vi "SPS-Variablen_nach_Cluster.vi"(8 "Fehler in":errorcluster, 11 "Cluster in":T2={"Initialisierung"={"Online?"=FALSE, "Grundpfad"=path "", "Kamera Oben"="", "IP-Adresse Flüssiglinse"="", "Flüssiglinse"=refnum, "Kamera Unten"="", "IP-Adresse SPS"="", "SPS-Verbindung"={"TCP Connection Ref"=refnum, "IP address"="", "timeout ms"=5000, "Connected?"=FALSE, "PLC Type"=enum."S7 1200", "Rack S7 400"=0, "Slot S7 400"=0, "PDU Size"=0, "connection semaphore"=refnum}, "IP-Adresse Lichtgitter"="", "Lichtgitter"=refnum, "Skalierungsfaktor"=0.0, "Bilder Oben"=[], "Bild Unten"=refnum, "Bild Ausschnitt Unten"=refnum}, "Einstellungen"={"Gesamtablauf gestartet"=FALSE, "i. O. Bilder speichern"=FALSE, "Bildspeicherung Offline"=FALSE, "Ausgewähltes Offline-Datum"="", "Ausgewähltes Offline-Teil"="", "Speicherpfad Bilder"=path ""}, "Artikeldaten"={"Artikelnummer"="", "Fertigungsauftrag"="", "Muster ISO"=refnum, "Belichtungszeit Referenzmarken"=0.0, "Fokus Referenzmarken"=0.0, "Belichtungszeit ISO"=0.0, "Fokus ISO"=0.0, "Belichtungszeit Unten"=0.0, "Kontaktanzahl"=0, "Aktueller Kontakt"=0, "Kontaktposition"={"x"=0.0, "y"=0.0}, "Winkel ISO"=0.0, "ISO-Muster nicht vorhanden"=FALSE}, "Werte Kamera Oben"={"Koordinatensystem"={"Punkt x-Achse"={"X"=0.0, "Y"=0.0}, "Ursprung"={"X"=0.0, "Y"=0.0}, "Punkt y-Achse"={"X"=0.0, "Y"=0.0}}, "Position Kontakt"={"x"=0.0, "y"=0.0}, "Winkel Kontakt"=0.0}, "Werte Kamera Unten"={"Prüfung Unten n. i. O."=FALSE}, "Werte Lichtgitter"={"Messwerte Referenzmarken"=[], "Mittelpunkt Referenzmarken"={"x"=0.0, "y"=0.0}, "Messwerte Kontakt"=[], "Offset"={"x"=0.0, "y"=0.0}}, "Rückmeldungen"={"Koordinaten ermittelt"=FALSE, "Vermessung Lichtgitter fertig"=FALSE, "Nachkontrolle Kamera Unten fertig"=FALSE}, "Fehler"={"Referenzen nicht gefunden"=FALSE, "Kontakt nicht gefunden"=FALSE, "Referenzen nicht in Lichtgitter"=FALSE, "Kontakt zu groß"=FALSE, "Kontakt zu klein"=FALSE}, "Statistik"={"Statistiken"=[]}, "Timer"={"Timer Start Position"=0, "Timer Start Lichtgitter"=0, "Timer Start Kamera Unten"=0}}) -> (0 "Fehler out":errorcluster, 1 "SPS OUT":T1, 2 "SPS IN":T10, 3 "Cluster out":T2={"Initialisierung"={"Online?"=FALSE, "Grundpfad"=path "", "Kamera Oben"="", "IP-Adresse Flüssiglinse"="", "Flüssiglinse"=refnum, "Kamera Unten"="", "IP-Adresse SPS"="", "SPS-Verbindung"={"TCP Connection Ref"=refnum, "IP address"="", "timeout ms"=5000, "Connected?"=FALSE, "PLC Type"=enum."S7 1200", "Rack S7 400"=0, "Slot S7 400"=0, "PDU Size"=0, "connection semaphore"=refnum}, "IP-Adresse Lichtgitter"="", "Lichtgitter"=refnum, "Skalierungsfaktor"=0.0, "Bilder Oben"=[], "Bild Unten"=refnum, "Bild Ausschnitt Unten"=refnum}, "Einstellungen"={"Gesamtablauf gestartet"=FALSE, "i. O. Bilder speichern"=FALSE, "Bildspeicherung Offline"=FALSE, "Ausgewähltes Offline-Datum"="", "Ausgewähltes Offline-Teil"="", "Speicherpfad Bilder"=path ""}, "Artikeldaten"={"Artikelnummer"="", "Fertigungsauftrag"="", "Muster ISO"=refnum, "Belichtungszeit Referenzmarken"=0.0, "Fokus Referenzmarken"=0.0, "Belichtungszeit ISO"=0.0, "Fokus ISO"=0.0, "Belichtungszeit Unten"=0.0, "Kontaktanzahl"=0, "Aktueller Kontakt"=0, "Kontaktposition"={"x"=0.0, "y"=0.0}, "Winkel ISO"=0.0, "ISO-Muster nicht vorhanden"=FALSE}, "Werte Kamera Oben"={"Koordinatensystem"={"Punkt x-Achse"={"X"=0.0, "Y"=0.0}, "Ursprung"={"X"=0.0, "Y"=0.0}, "Punkt y-Achse"={"X"=0.0, "Y"=0.0}}, "Position Kontakt"={"x"=0.0, "y"=0.0}, "Winkel Kontakt"=0.0}, "Werte Kamera Unten"={"Prüfung Unten n. i. O."=FALSE}, "Werte Lichtgitter"={"Messwerte Referenzmarken"=[], "Mittelpunkt Referenzmarken"={"x"=0.0, "y"=0.0}, "Messwerte Kontakt"=[], "Offset"={"x"=0.0, "y"=0.0}}, "Rückmeldungen"={"Koordinaten ermittelt"=FALSE, "Vermessung Lichtgitter fertig"=FALSE, "Nachkontrolle Kamera Unten fertig"=FALSE}, "Fehler"={"Referenzen nicht gefunden"=FALSE, "Kontakt nicht gefunden"=FALSE, "Referenzen nicht in Lichtgitter"=FALSE, "Kontakt zu groß"=FALSE, "Kontakt zu klein"=FALSE}, "Statistik"={"Statistiken"=[]}, "Timer"={"Timer Start Position"=0, "Timer Start Lichtgitter"=0, "Timer Start Kamera Unten"=0}})   [LabVIEW 2024]
doc: "Bündelt die Globalen Variablen von der SPS in Cluster und gibt diese aus."
uses:
  Cluster_SPS_IN.ctl
  Cluster.ctl
  Kontaktmontagemodul.exe/1abvi3w/vi.lib/userDefined/High Color/IMAQdx.ctl
  Kontaktmontagemodul.exe/1abvi3w/vi.lib/DATA AHEAD/SP7/typedefs/S7 Connection.ctl
  Kontaktmontagemodul.exe/1abvi3w/vi.lib/DATA AHEAD/SP7/typedefs/PLC Type.ctl
  Kontaktmontagemodul.exe/1abvi3w/vi.lib/vision/Image Controls.llb/IMAQ Image.ctl
  Koordinatensystem.ctl
  Statistik.ctl
  Cluster_SPS_OUT.ctl
  Globale Variablen.vi
  Kontaktmontagemodul.exe/1abvi3w/vi.lib/DATA AHEAD/SP7/SP7.lvlib
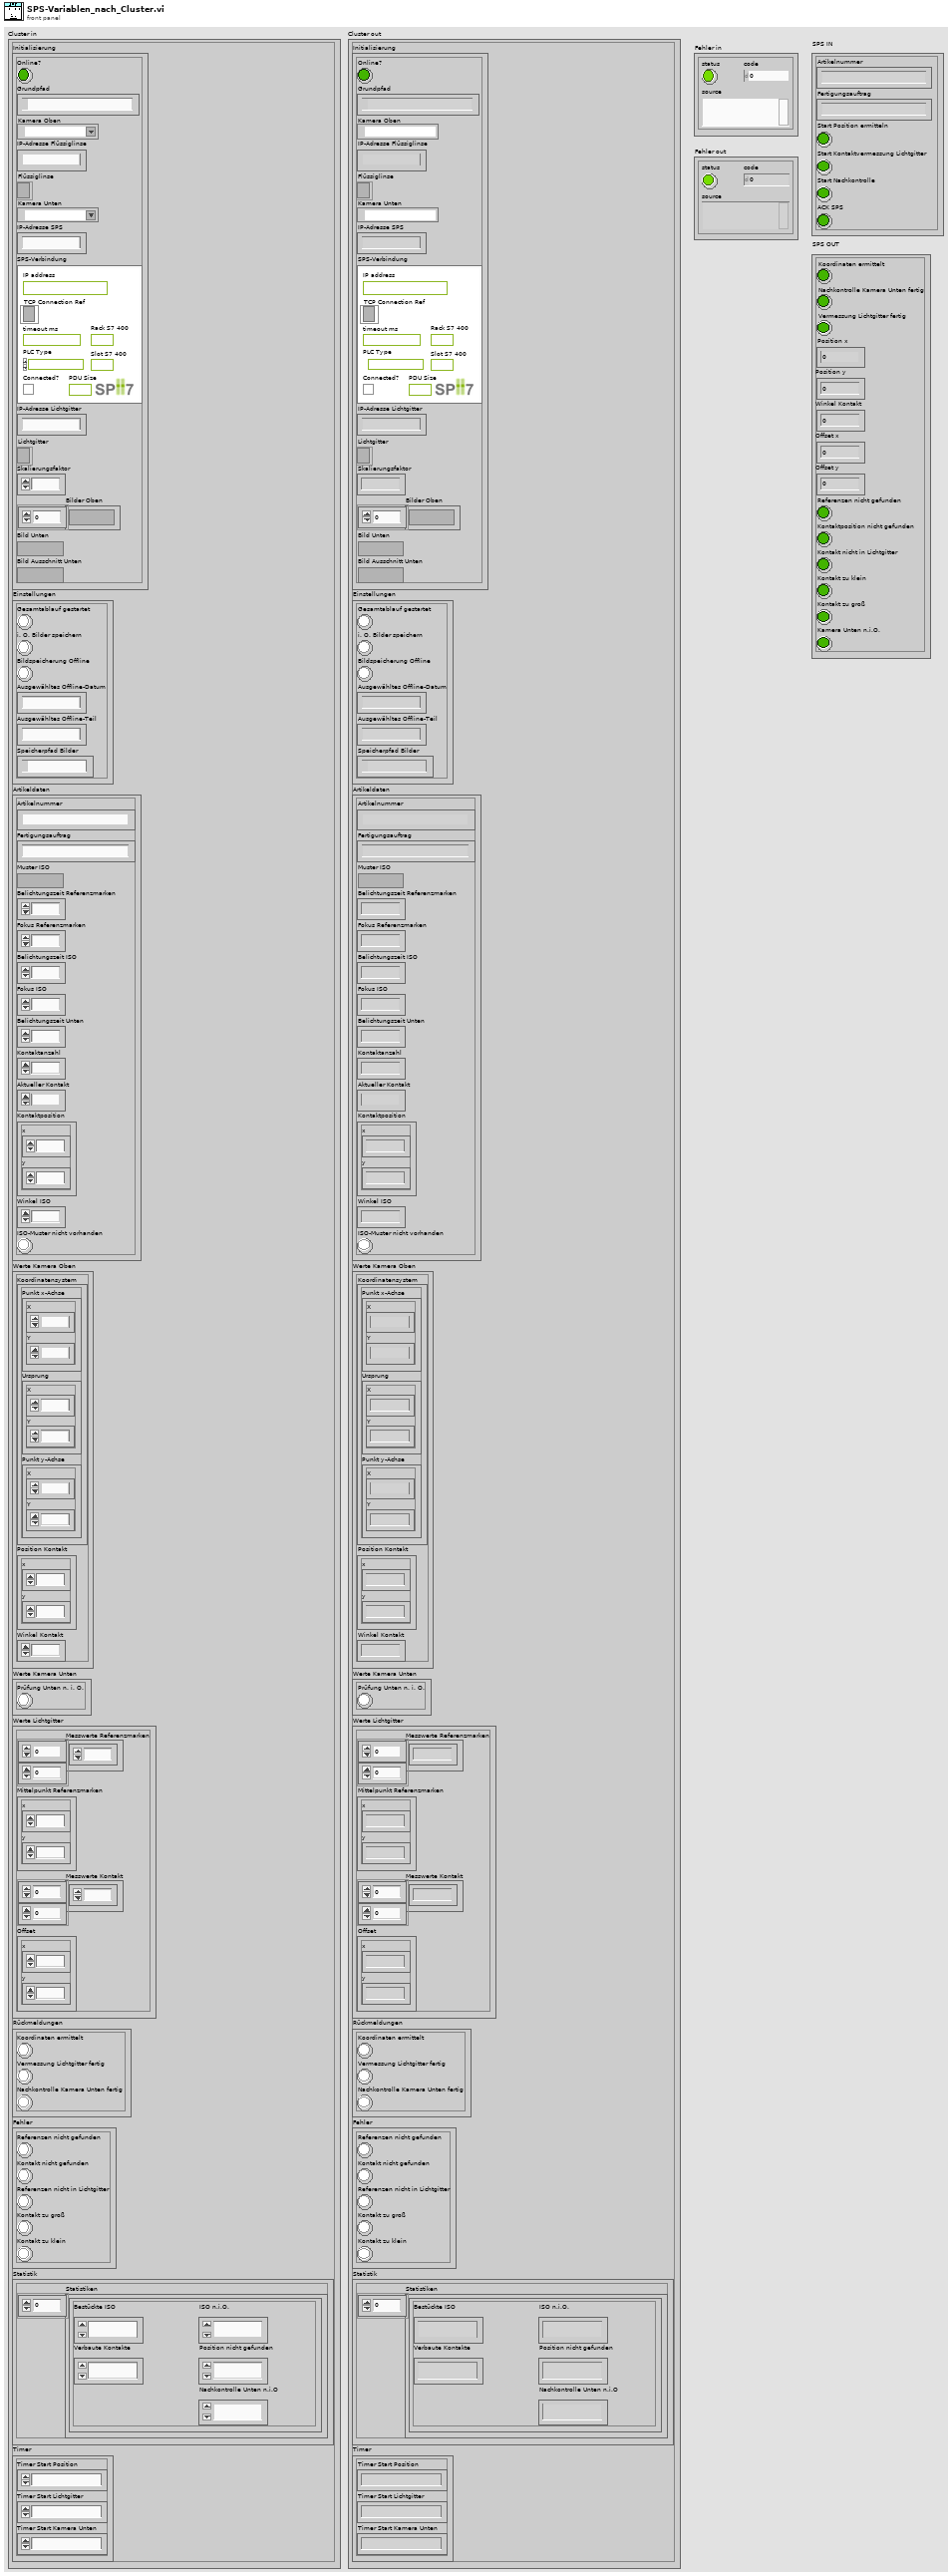
[diagram p1: front panel]
types:
  T1 = typedef "Cluster_SPS_OUT.ctl" = cluster{"Koordinaten ermittelt":bool, "Nachkontrolle Kamera Unten fertig":bool, "Vermessung Lichtgitter fertig":bool, "Position x":dbl, "Position y":dbl, "Winkel Kontakt":dbl, "Offset x":dbl, "Offset y":dbl, "Referenzen nicht gefunden":bool, "Kontaktposition nicht gefunden":bool, "Kontakt nicht in Lichtgitter":bool, "Kontakt zu klein":bool, "Kontakt zu groß":bool, "Kamera Unten n.i.O.":bool}
  T2 = typedef "Cluster.ctl" = cluster{"Initialisierung":cluster{"Online?":bool, "Grundpfad":path, "Kamera Oben":T3, "IP-Adresse Flüssiglinse":string, "Flüssiglinse":refnum<k5>, "Kamera Unten":T3, "IP-Adresse SPS":string, "SPS-Verbindung":T4, "IP-Adresse Lichtgitter":string, "Lichtgitter":refnum<k5>, "Skalierungsfaktor":dbl, "Bilder Oben":T7[], "Bild Unten":T7, "Bild Ausschnitt Unten":T7}, "Einstellungen":cluster{"Gesamtablauf gestartet":bool, "i. O. Bilder speichern":bool, "Bildspeicherung Offline":bool, "Ausgewähltes Offline-Datum":string, "Ausgewähltes Offline-Teil":string, "Speicherpfad Bilder":path}, "Artikeldaten":cluster{"Artikelnummer":string, "Fertigungsauftrag":string, "Muster ISO":T7, "Belichtungszeit Referenzmarken":dbl, "Fokus Referenzmarken":dbl, "Belichtungszeit ISO":dbl, "Fokus ISO":dbl, "Belichtungszeit Unten":dbl, "Kontaktanzahl":u32, "Aktueller Kontakt":i16, "Kontaktposition":cluster{"x":sgl, "y":sgl}, "Winkel ISO":sgl, "ISO-Muster nicht vorhanden":bool}, "Werte Kamera Oben":cluster{"Koordinatensystem":T8, "Position Kontakt":cluster{"x":dbl, "y":dbl}, "Winkel Kontakt":dbl}, "Werte Kamera Unten":cluster{"Prüfung Unten n. i. O.":bool}, "Werte Lichtgitter":cluster{"Messwerte Referenzmarken":dbl[][], "Mittelpunkt Referenzmarken":cluster{"x":dbl, "y":dbl}, "Messwerte Kontakt":dbl[][], "Offset":cluster{"x":dbl, "y":dbl}}, "Rückmeldungen":cluster{"Koordinaten ermittelt":bool, "Vermessung Lichtgitter fertig":bool, "Nachkontrolle Kamera Unten fertig":bool}, "Fehler":cluster{"Referenzen nicht gefunden":bool, "Kontakt nicht gefunden":bool, "Referenzen nicht in Lichtgitter":bool, "Kontakt zu groß":bool, "Kontakt zu klein":bool}, "Statistik":cluster{"Statistiken":T9[]}, "Timer":cluster{"Timer Start Position":u32, "Timer Start Lichtgitter":u32, "Timer Start Kamera Unten":u32}}
  T3 = typedef "IMAQdx.ctl" = refnum<k21>
  T4 = typedef "SP7.lvlib/S7 Connection.ctl" = cluster{"TCP Connection Ref":refnum<k5>, "IP address":string, "timeout ms":i32, "Connected?":bool, "PLC Type":T5, "Rack S7 400":u8, "Slot S7 400":u8, "PDU Size":u16, "connection semaphore":T6}
  T5 = typedef "SP7.lvlib/PLC Type.ctl" = enum16{"S7 200", "S7 300/400", "S7 1200", "S7 1500", "LOGO!8"}
  T6 = typedef "Semaphore RefNum" = refnum<k1>
  T7 = typedef "IMAQ Image.ctl" = refnum<image>
  T8 = typedef "Koordinatensystem.ctl" = cluster{"Punkt x-Achse":cluster{"X":sgl, "Y":sgl}, "Ursprung":cluster{"X":sgl, "Y":sgl}, "Punkt y-Achse":cluster{"X":sgl, "Y":sgl}}
  T9 = typedef "Statistik.ctl" = cluster{"Bestückte ISO":u32, "Verbaute Kontakte":u32, "ISO n.i.O.":u32, "Nachkontrolle Unten n.i.O":u32, "Position nicht gefunden":u32}
  T10 = typedef "Cluster_SPS_IN.ctl" = cluster{"Artikelnummer":string, "Fertigungsauftrag":string, "Start Position ermitteln":bool, "Start Kontaktvermessung Lichtgitter":bool, "Start Nachkontrolle":bool, "ACK SPS":bool}
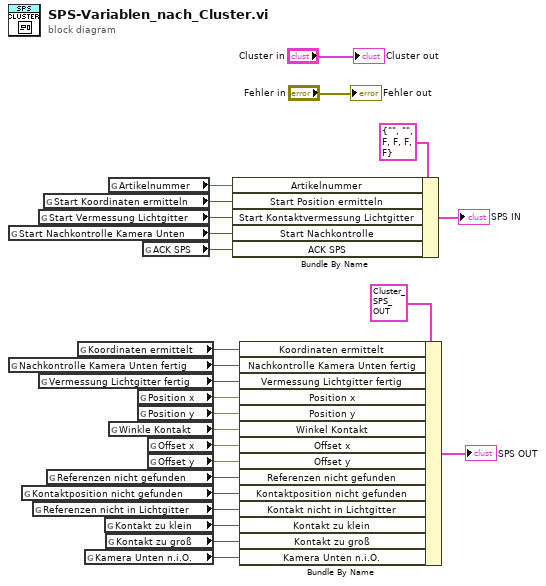
[diagram p0: block diagram]
diagram:
  n1 = global read "Globale Variablen.vi" "Start Nachkontrolle Kamera Unten"() -> (w18:bool)
  n2 = global read "Globale Variablen.vi" "Nachkontrolle Kamera Unten fertig"() -> (w14:bool)
  n3 = global read "Globale Variablen.vi" "Kontaktposition nicht gefunden"() -> (w6:bool)
  n4 = global read "Globale Variablen.vi" "Referenzen nicht in Lichtgitter"() -> (w5:bool)
  n5 = global read "Globale Variablen.vi" "Start Vermessung Lichtgitter"() -> (w19:bool)
  n6 = global read "Globale Variablen.vi" "Vermessung Lichtgitter fertig"() -> (w13:bool)
  n7 = global read "Globale Variablen.vi" "Start Koordinaten ermitteln"() -> (w24:bool)
  n8 = global read "Globale Variablen.vi" "Referenzen nicht gefunden"() -> (w7:bool)
  n9 = global read "Globale Variablen.vi" "Koordinaten ermittelt"() -> (w15:bool)
  n10 = global read "Globale Variablen.vi" "Kamera Unten n.i.O."() -> (w1:bool)
  n11 = global read "Globale Variablen.vi" "Kontakt zu klein"() -> (w4:bool)
  n12 = global read "Globale Variablen.vi" "Kontakt zu groß"() -> (w3:bool)
  n13 = global read "Globale Variablen.vi" "Artikelnummer"() -> (w20:string)
  n14 = global read "Globale Variablen.vi" "Winkle Kontakt"() -> (w10:dbl)
  n15 = global read "Globale Variablen.vi" "Position x"() -> (w12:dbl)
  n16 = global read "Globale Variablen.vi" "Position y"() -> (w11:dbl)
  n17 = global read "Globale Variablen.vi" "ACK SPS"() -> (w2:bool)
  n18 = global read "Globale Variablen.vi" "Offset x"() -> (w9:dbl)
  n19 = global read "Globale Variablen.vi" "Offset y"() -> (w8:dbl)
  n20 = Bundle By Name(cluster=T10 {"Artikelnummer"="", "Fertigungsauftrag"="", "Start Position ermitteln"=FALSE, "Start Kontaktvermessung Lichtgitter"=FALSE, "Start Nachkontrolle"=FALSE, "ACK SPS"=FALSE} ("SPS IN"), "Artikelnummer"=w20, "Start Position ermitteln"=w24, "Start Kontaktvermessung Lichtgitter"=w19, "Start Nachkontrolle"=w18, "ACK SPS"=w2) -> (→"SPS IN":T10)
  n21 = Bundle By Name(cluster=T1 {"Koordinaten ermittelt"=FALSE, "Nachkontrolle Kamera Unten fertig"=FALSE, "Vermessung Lichtgitter fertig"=FALSE, "Position x"=0.0, "Position y"=0.0, "Winkel Kontakt"=0.0, "Offset x"=0.0, "Offset y"=0.0, "Referenzen nicht gefunden"=FALSE, "Kontaktposition nicht gefunden"=FALSE, "Kontakt nicht in Lichtgitter"=FALSE, "Kontakt zu klein"=FALSE, "Kontakt zu groß"=FALSE, "Kamera Unten n.i.O."=FALSE} ("SPS OUT"), "Koordinaten ermittelt"=w15, "Nachkontrolle Kamera Unten fertig"=w14, "Vermessung Lichtgitter fertig"=w13, "Position x"=w12, "Position y"=w11, "Winkel Kontakt"=w10, "Offset x"=w9, "Offset y"=w8, "Referenzen nicht gefunden"=w7, "Kontaktposition nicht gefunden"=w6, "Kontakt nicht in Lichtgitter"=w5, "Kontakt zu klein"=w4, "Kontakt zu groß"=w3, "Kamera Unten n.i.O."=w1) -> (→"SPS OUT":T1)
  "Fehler out" <- "Fehler in"
  "Cluster out" <- "Cluster in"
